vi "AxisSpace.vi"() -> ()   [LabVIEW 2009]
uses:
  typedefs/AxisSpaceCfg.ctl
  typedefs/AxisCfg.ctl
panel:
  in  "Axis Space":T1=[{"Addr"=88, "Conv Factor"=0.0, "Forward Limit"=0.0, "Reverse Limit"=0.0, "Enable Limits"=FALSE}, {"Addr"=89, "Conv Factor"=0.0, "Forward Limit"=0.0, "Reverse Limit"=0.0, "Enable Limits"=FALSE}, {"Addr"=90, "Conv Factor"=0.0, "Forward Limit"=0.0, "Reverse Limit"=0.0, "Enable Limits"=FALSE}, {"Addr"=255, "Conv Factor"=0.0, "Forward Limit"=0.0, "Reverse Limit"=0.0, "Enable Limits"=FALSE}]
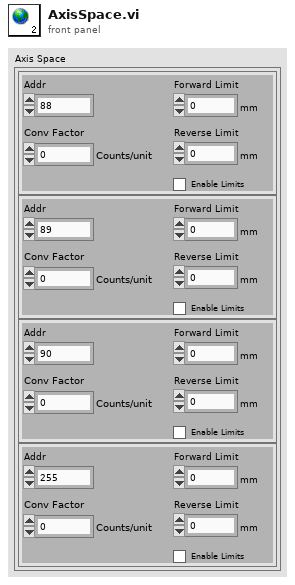
[diagram p1: front panel]
types:
  T1 = typedef "AxisSpaceCfg.ctl" = T2[]
  T2 = typedef "AxisCfg.ctl" = cluster{"Addr":u8, "Conv Factor":dbl, "Forward Limit":dbl, "Reverse Limit":dbl, "Enable Limits":bool}
diagram:
